vi "NI VeriStand - Visually Update the System Explorer Tree.vi"(8 "error in (no error)":errorcluster, 10 "Action":T1=7 items=["Refresh (Add)"=5, "Refresh (Repopulate node)"=7, "Refresh (Delete)"=9], 11 "Node IDs":u64[](array[numeric])) -> (0 "error out":errorcluster)   [LabVIEW 2017, in "Import Export.lvlib"]
doc: "***This VI is not officially supported by National Instruments*** due to CAR 317524"
uses:
  Import Export.lvlib
  System Explorer Action.ctl
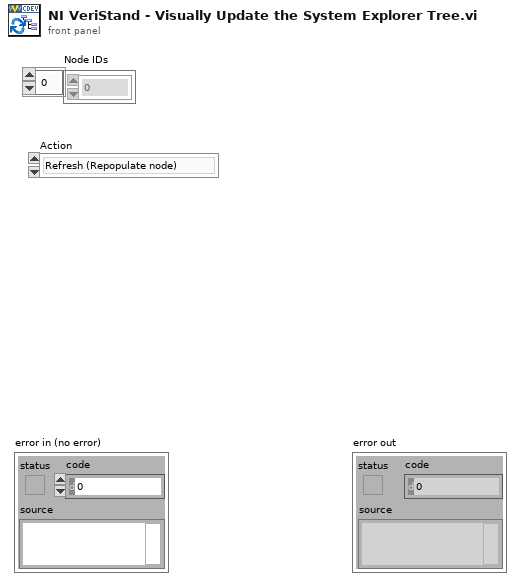
[diagram p1: front panel]
types:
  T1 = typedef "Import Export.lvlib/System Explorer Action.ctl" = u16
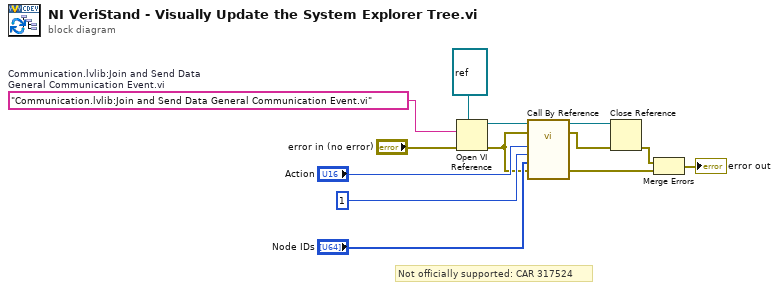
[diagram p0: block diagram]
diagram:
  w13 = "Communication.lvlib:Join and Send Data General Communication Event.vi"  # Communication.lvlib:Join and Send Data General Communication Event.vi
  # "Not officially supported: CAR 317524"
  n1 = Open VI Reference(type specifier VI Refnum (for type only)=refnum<vi> refnum, vi path=w13, error in (no error)="error in (no error)") -> (vi reference=w3:refnum<vi>, error out=w2:errorcluster)  [unwired: 3 in]
  n2 = call-by-ref "?"(reference=w3, error in=w2, 8:"error in (no error)"=w2, "Data in"="Node IDs", "Listener"=1, "Action"="Action") -> (reference out=w6:refnum<vi>, error out=w7:errorcluster, 0:"error out"=w4:errorcluster)  [unwired: 6 in, 1 out]
  n3 = Close Reference(reference=w6, error in (no error)=w7) -> (error out=w5:errorcluster)
  n4 = Merge Errors(w5, w4) -> (→"error out":errorcluster)
